vi "Sub.vi"(8 "error in":errorcluster, 9 "queue group":string, 10 "subject":string, 11 "NATS Client":refnum<class "NATS Client.lvclass">) -> (0 "error out":errorcluster, 3 "NATS Subscription":refnum<class "NATS Subscription.lvclass">)   [LabVIEW 2020, in "NATS Subscription.lvlib" / "NATS Subscription.lvclass"]
doc: "Creates and registers a subscription with the NATS Client."
uses:
  NATS Subscription.lvclass
  NATS Client/NATS Client.lvclass
  NATS Subscription.lvclass/NATS Subscription.ctl
  <vilib>/NATS/NATS Core/Controls/msg type.ctl
  <vilib>/NATS/NATS Core/NATS Core.lvlib
  <vilib>/NATS/NATS Core/Controls/nats message.ctl
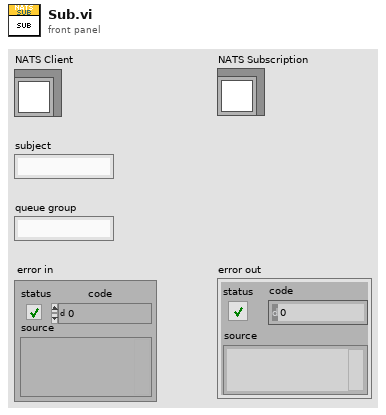
[diagram p1: front panel]
types:
  T1 = typedef "NATS Core.lvlib/nats message.ctl" = cluster{"subject":string, "payload":string, "sub id":string, "reply-to":string, "headers":string, "type":T2, "received":timestamp}
  T2 = typedef "NATS Core.lvlib/msg type.ctl" = enum16{"Undefined", "MSG", "HMSG", "+OK", "PING", "PONG", "-ERR", "INFO"}
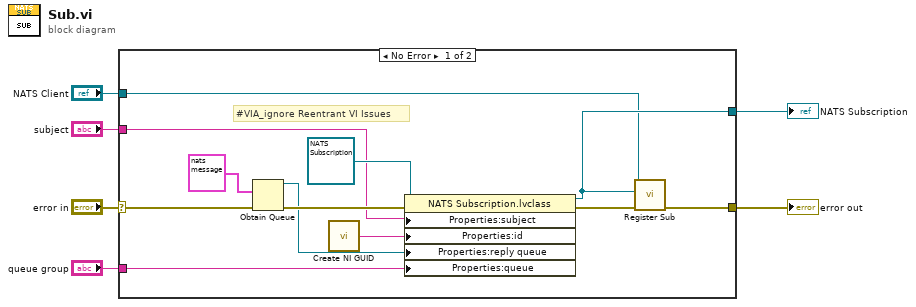
[diagram p0: block diagram]
diagram:
  n1 = case shown="No Error" "error in" {
    selector: "error in" -> [w18 w19]
    tunnel: "subject" -> [w13 _]
    tunnel: [w16 w19] -> w5
    tunnel: [w9 _] -> w3
    tunnel: "NATS Client" -> [w8 _]
    tunnel: "queue group" -> [w7 _]
    frame No Error {
      # "#VIA_ignore Reentrant VI Issues"
      n2 = Obtain Queue(element data type=T1 {"subject"="", "payload"="", "sub id"="", "reply-to"="", "headers"="", "type"=enum."Undefined", "received"=timestamp(0 s since 1904-01-01)} ("nats message"), error in (no error)=w18) -> (queue out=w10:refnum<queue>, error out=w17:errorcluster)  [unwired: 3 in, 1 out]
      n3 = call <vilib>:"Create NI GUID.vi"() -> ("NI GUID"=w12:string)
      n4 = property class="NATS Subscription.lvclass"(reference=refnum<class "NATS Subscription.lvclass"> refnum ("NATS Core.lvlib:NATS Subscription.lvclass"), error in=w17, "Properties:subject"=w13, "Properties:id"=w12, "Properties:reply queue"=w10, "Properties:queue"=w7) -> (reference out=w9:refnum<class "NATS Subscription.lvclass">, error out=w15:errorcluster)
      n5 = call "Register Sub.vi"("error in"=w15, "NATS Subscription"=w9, "NATS Client in"=w8) -> ("error out"=w16:errorcluster)  [unwired: 7 in, 1 out]
    }
    frame Error {
    }
  }
  "error out" <- w5
  "NATS Subscription" <- w3
